vi "ActionVIOnCompile.vi"(8 "error in (no error)":errorcluster, 11 "Device Item Ref in":T1 format="%.0x") -> (0 "error out":errorcluster)   [LabVIEW 2015, in "DMM-SWITCH-ScanList System Explorer.lvlib"]
uses:
  DMM-SWITCH-ScanList System Explorer.lvlib
  <vilib>/NI Veristand/Custom Device API/Custom Device Item Ref.ctl
  Shared/Compiled.Settings
  Engine/TypeDefs/DMM-Switch Configuration.ctl
  <instrlib>/niDMM/nidmm.llb/niDMM Function.ctl
  <instrlib>/niDMM/nidmm.llb/niDMM Resolution in Digits.ctl
  <instrlib>/niSwitch/niSwitch.LLB/niSwitch Topologies.ctl
  <instrlib>/niSwitch/niSwitch.LLB/niSwitch Trigger Input.ctl
  <instrlib>/niSwitch/niSwitch.LLB/niSwitch Scan Advanced Output.ctl
  <instrlib>/niDMM/nidmm.llb/niDMM Measurement Complete.ctl
  <instrlib>/niDMM/nidmm.llb/niDMM Trigger.ctl
  <vilib>/NI Veristand/Custom Device Tools/Custom Device Utility Library/NI VeriStand - Search for Item by Name.vi
  <vilib>/NI Veristand/Custom Device API/Set Item Property (Variant).vi
  <vilib>/NI Veristand/Custom Device API/Custom Device API.lvlib
  Engine/DMM-SWITCH-ScanList Engine.lvlib
  <vilib>/NI Veristand/Custom Device Tools/Custom Device Utility Library/Custom Device Utility Library.lvlib
  <vilib>/addons/Inline Async API/_Data Access System Explorer/Data Access System Explorer.lvlib
  Shared/DMM-SWITCH-ScanList Shared.lvlib
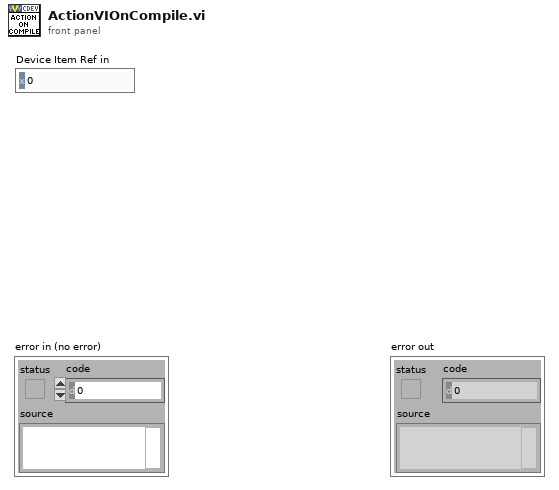
[diagram p1: front panel]
types:
  T1 = typedef "Custom Device API.lvlib/Custom Device Item Ref.ctl" = u64
  T2 = typedef "DMM-SWITCH-ScanList Engine.lvlib/DMM-Switch Configuration.ctl" = cluster{"DMM Resource Name":string, "DMM Measurement":T3, "DMM Resolution in Digits":T4, "DMM Range [EU]":dbl, "Switch Resource Name":string, "Switch Topology":T5, "Switch Scan List":string, "Switch Trigger Source":T6, "Switch Scan Advanced Output":T7, "DMM Measurement Complete":T8, "DMM Trigger Source":T9, "# of Channels":u32, "Group CH Names - Configuration":string, "Group CH Names - Input Channels":string, "Group CH Names - Measurement Channels":string, "Group CH Names - Runtime Status":string}
  T3 = typedef "niDMM Function.ctl" = enum16{"DC Volts", "AC Volts", "DC Current", "AC Current", "2-wire Resistance", "4-wire Resistance", "Diode", "Frequency", "Period", "AC Volts DC Coupled", "Capacitance", "Inductance", "Temperature"}
  T4 = typedef "niDMM Resolution in Digits.ctl" = dbl
  T5 = typedef "niSwitch Topologies.ctl" = string
  T6 = typedef "niSwitch Trigger Input.ctl" = enum16{"Immediate", "External", "TTL0", "TTL1", "TTL2", "TTL3", "TTL4", "TTL5", "TTL6", "TTL7", "ECL0", "ECL1", "PXI Star", "Software Trigger Function", "Rear Connector", "Front Connector", "Rear Connector of Module 1", "Rear Connector of Module 2", "Rear Connector of Module 3", "Rear Connector of Module 4", "Rear Connector of Module 5", "Rear Connector of Module 6", "Rear Connector of Module 7", "Rear Connector of Module 8", "Rear Connector of Module 9", "Rear Connector of Module 10", "Rear Connector of Module 11", "Rear Connector of Module 12", "Front Connector of Module 1", "Front Connector of Module 2", "Front Connector of Module 3", "Front Connector of Module 4", "Front Connector of Module 5", "Front Connector of Module 6", "Front Connector of Module 7", "Front Connector of Module 8", "Front Connector of Module 9", "Front Connector of Module 10", "Front Connector of Module 11", "Front Connector of Module 12"}
  T7 = typedef "niSwitch Scan Advanced Output.ctl" = enum16{"None", "External", "TTL0", "TTL1", "TTL2", "TTL3", "TTL4", "TTL5", "TTL6", "TTL7", "ECL0", "ECL1", "PXI Star", "Rear Connector", "Front Connector", "Rear Connector Module 1", "Rear Connector Module 2", "Rear Connector Module 3", "Rear Connector Module 4", "Rear Connector Module 5", "Rear Connector Module 6", "Rear Connector Module 7", "Rear Connector Module 8", "Rear Connector Module 9", "Rear Connector Module 10", "Rear Connector Module 11", "Rear Connector Module 12", "Front Connector Module 1", "Front Connector Module 2", "Front Connector Module 3", "Front Connector Module 4", "Front Connector Module 5", "Front Connector Module 6", "Front Connector Module 7", "Front Connector Module 8", "Front Connector Module 9", "Front Connector Module 10", "Front Connector Module 11", "Front Connector Module 12"}
  T8 = typedef "niDMM Measurement Complete.ctl" = enum16{"None", "External", "TTL 0", "TTL 1", "TTL 2", "TTL 3", "TTL 4", "TTL 5", "TTL 6", "TTL 7", "LBR Trig 0"}
  T9 = typedef "niDMM Trigger.ctl" = enum16{"Immediate", "External", "TTL 0", "TTL 1", "TTL 2", "TTL 3", "TTL 4", "TTL 5", "TTL 6", "Software", "TTL 7", "PXI Star", "LBR Trig 1", "Aux Trig 1"}
  T10 = typedef "DMM-SWITCH-ScanList Shared.lvlib/Compiled.Settings" = cluster{"Name":string, "DMM-Switch Configuration":T2}
  T11 = enum16{"Output/Write", "Input/Read", "Input/ReadWrite"}
  T12 = cluster{"Name":string, "Type":enum16{"Output/Write", "Input/Read", "Input/ReadWrite"}, "VS Refs":T1[]}
  T13 = typedef "Custom Device API.lvlib/Custom Device Item Info.ctl" = cluster{"Name":string, "Is Channel":bool, "GUID":string, "Is Waveform":bool}
  T14 = cluster{"Name":string, "Type":enum16{"Output/Write", "Input/Read", "Input/ReadWrite"}, "VS Refs":T1[]}[]
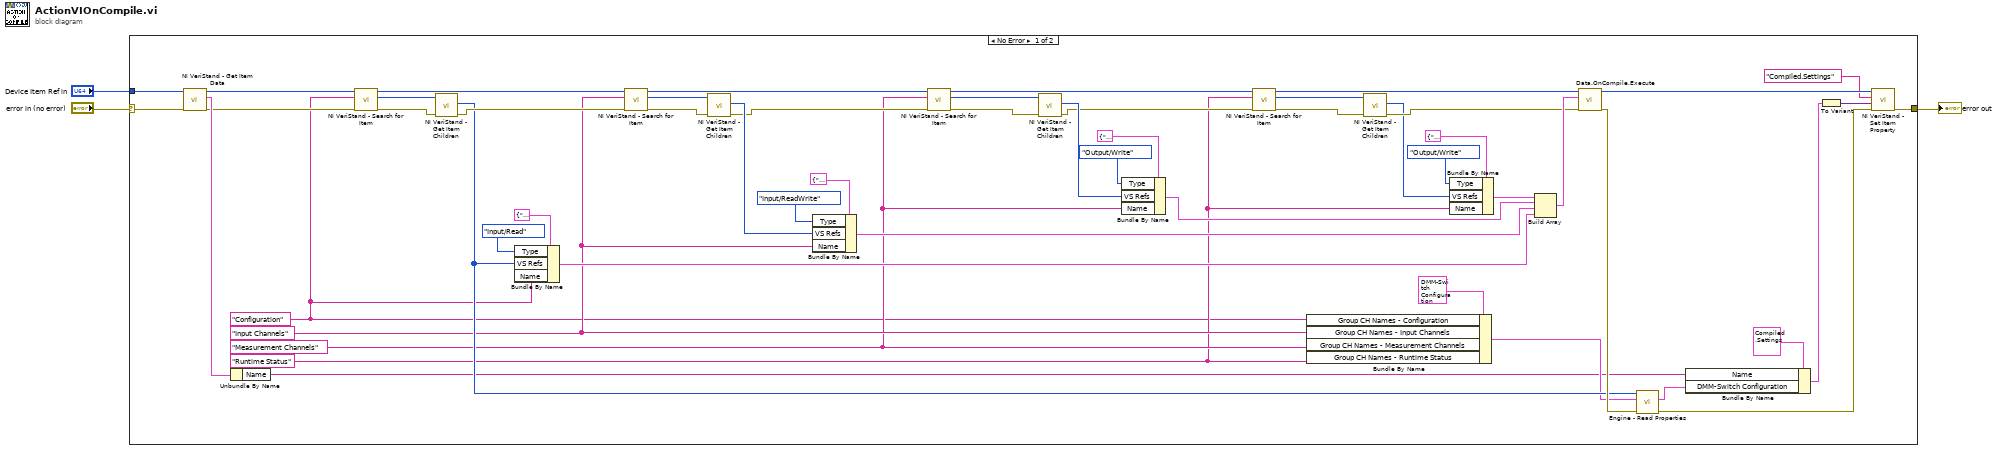
[diagram p0: block diagram]
diagram:
  n1 = case shown="No Error" "error in (no error)" {
    selector: "error in (no error)" -> [w56 w58]
    tunnel: "Device Item Ref in" -> [w57 _]
    tunnel: [w11 w58] -> w1
    frame No Error {
      w12 = "Runtime Status" ("Group Ch - Runtime Status")
      w13 = "Measurement Channels" ("Group Ch - Measurement Channels")
      w14 = "Input Channels" ("Group Ch - Input Channels")
      w10 = "Configuration" ("Group Ch - Configuration")
      n2 = call <vilib>:"NI VeriStand - Get Item Data.vi"("error in (no error)"=w56, "Item Ref in"=w57) -> ("error out"=w33:errorcluster, "Item Info"=w36:T13, "Item Ref out"=w55:T1)  [unwired: 6 in, 1 out]
      n3 = Unbundle By Name(w36) -> ("Name"=w6:string)
      n4 = call-poly <vilib>:"NI VeriStand - Search for Item.vi"("error in"=w33, "Item Name"=w10, "Section Ref in"=w55) -> ("error out"=w32:errorcluster, "Item Ref"=w54:T1, "Section Ref out"=w43:T1)  [unwired: 5 in, 1 out]
      n5 = call <vilib>:"NI VeriStand - Get Item Children.vi"("error in (no error)"=w32, "Item Ref in"=w54) -> ("error out"=w42:errorcluster, "Child Refs"=w29:T1[])  [unwired: 6 in, 2 out]
      n6 = Bundle By Name(cluster=T12 {"Name"="", "Type"=enum."Output/Write", "VS Refs"=[]} ("Group"), "Type"=T11."Input/Read", "VS Refs"=w29, "Name"=w10) -> (w37:T12)
      n7 = call-poly <vilib>:"NI VeriStand - Search for Item.vi"("error in"=w42, "Item Name"=w14, "Section Ref in"=w43) -> ("error out"=w45:errorcluster, "Item Ref"=w46:T1, "Section Ref out"=w40:T1)  [unwired: 5 in, 1 out]
      n8 = call <vilib>:"NI VeriStand - Get Item Children.vi"("error in (no error)"=w45, "Item Ref in"=w46) -> ("error out"=w41:errorcluster, "Child Refs"=w47:T1[])  [unwired: 6 in, 2 out]
      n9 = Bundle By Name(cluster=T12 {"Name"="", "Type"=enum."Output/Write", "VS Refs"=[]} ("Group"), "Type"=T11."Input/ReadWrite", "VS Refs"=w47, "Name"=w14) -> (w38:T12)
      n10 = call-poly <vilib>:"NI VeriStand - Search for Item.vi"("error in"=w41, "Item Name"=w13, "Section Ref in"=w40) -> ("error out"=w17:errorcluster, "Item Ref"=w25:T1, "Section Ref out"=w20:T1)  [unwired: 5 in, 1 out]
      n11 = call <vilib>:"NI VeriStand - Get Item Children.vi"("error in (no error)"=w17, "Item Ref in"=w25) -> ("error out"=w18:errorcluster, "Child Refs"=w26:T1[])  [unwired: 6 in, 2 out]
      n12 = Bundle By Name(cluster=T12 {"Name"="", "Type"=enum."Output/Write", "VS Refs"=[]} ("Group"), "Type"=T11."Output/Write", "VS Refs"=w26, "Name"=w13) -> (w15:T12)
      n13 = call-poly <vilib>:"NI VeriStand - Search for Item.vi"("error in"=w18, "Item Name"=w12, "Section Ref in"=w20) -> ("error out"=w24:errorcluster, "Item Ref"=w21:T1, "Section Ref out"=w39:T1)  [unwired: 5 in, 1 out]
      n14 = Bundle By Name(cluster=T2 {"DMM Resource Name"="", "DMM Measurement"=enum."DC Volts", "DMM Resolution in Digits"=0.0, "DMM Range [EU]"=0.0, "Switch Resource Name"="", "Switch Topology"="", "Switch Scan List"="", "Switch Trigger Source"=enum."Immediate", "Switch Scan Advanced Output"=enum."None", "DMM Measurement Complete"=enum."None", "DMM Trigger Source"=enum."Immediate", "# of Channels"=0, "Group CH Names - Configuration"="", "Group CH Names - Input Channels"="", "Group CH Names - Measurement Channels"="", "Group CH Names - Runtime Status"=""} ("DMM-Switch Configuration Out"), "Group CH Names - Configuration"=w10, "Group CH Names - Input Channels"=w14, "Group CH Names - Measurement Channels"=w13, "Group CH Names - Runtime Status"=w12) -> (w9:T2)
      n15 = call <vilib>:"NI VeriStand - Get Item Children.vi"("error in (no error)"=w24, "Item Ref in"=w21) -> ("error out"=w31:errorcluster, "Child Refs"=w22:T1[])  [unwired: 6 in, 2 out]
      n16 = Bundle By Name(cluster=T12 {"Name"="", "Type"=enum."Output/Write", "VS Refs"=[]} ("Group"), "Type"=T11."Output/Write", "VS Refs"=w22, "Name"=w12) -> (w16:T12)
      n17 = Build Array(w16, w15, w38, w37) -> (w49:T14)
      n18 = call <vilib>:"Data.OnCompile.Execute.vi"("error in"=w31, "VS Ref Groups"=w49, "Custom Device Ref"=w39) -> ("error out"=w30:errorcluster, "Custom Device Ref"=w53:T1)  [unwired: 7 in]
      n19 = call "Engine - Read Properties.vi"("error in (no error)"=w30, "DMM-Switch Configuration In"=w9, "Specified Channel Ref List In"=w29) -> ("error out"=w34:errorcluster, "DMM-Switch Configuration Out"=w5:T2)  [unwired: 6 in, 1 out]
      n20 = Bundle By Name(cluster=T10 {"Name"="", "DMM-Switch Configuration"={"DMM Resource Name"="", "DMM Measurement"=enum."DC Volts", "DMM Resolution in Digits"=6.5, "DMM Range [EU]"=10.0, "Switch Resource Name"="", "Switch Topology"="2503/2-Wire 24x1 Mux", "Switch Scan List"="ab0->com0 & com0->ch0:2;", "Switch Trigger Source"=enum."TTL0", "Switch Scan Advanced Output"=enum."TTL1", "DMM Measurement Complete"=enum."TTL 0", "DMM Trigger Source"=enum."TTL 1", "# of Channels"=0, "Group CH Names - Configuration"="", "Group CH Names - Input Channels"="", "Group CH Names - Measurement Channels"="", "Group CH Names - Runtime Status"=""}} ("Compiled.Settings"), "Name"=w6, "DMM-Switch Configuration"=w5) -> (w4:T10)
      n21 = To Variant(anything=w4) -> (Variant=w35:variant)
      n22 = call-poly <vilib>:"NI VeriStand - Set Item Property.vi"("error in (no error)"=w34, "Value"=w35, "Property Name"="Compiled.Settings", "Item Ref in"=w53) -> ("error out"=w11:errorcluster)  [unwired: 5 in, 2 out]
    }
    frame Error {
    }
  }
  "error out" <- w1
